vi "meth.PushErrorState.vi"(0 "class.GLue in":refnum<class "class.GLue.lvclass">, 11 "error in (no error)":errorcluster) -> (4 "class.GLue out":refnum<class "class.GLue.lvclass">, 8 "NumPushed":i32, 15 "error out":errorcluster)   [LabVIEW 2014, in "GLue.lvlib" / "class.GLue.lvclass"]
uses:
  class.GLue.lvclass
  class.GLue.lvclass/class.GLue.ctl
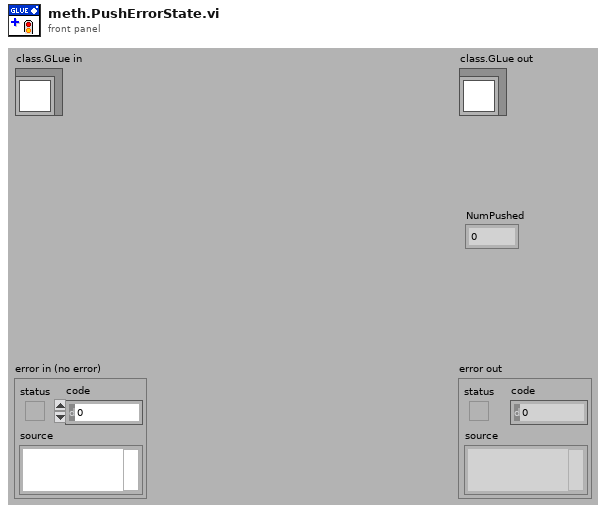
[diagram p1: front panel]
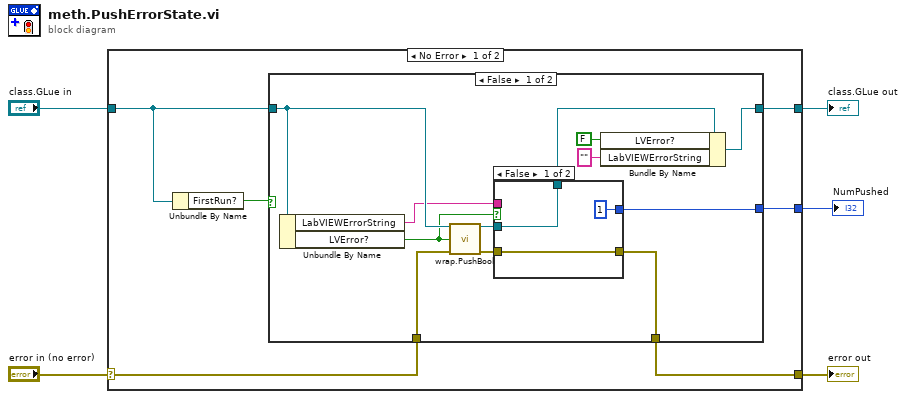
[diagram p0: block diagram]
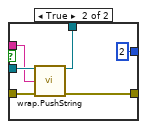
[diagram p2: hidden frame]
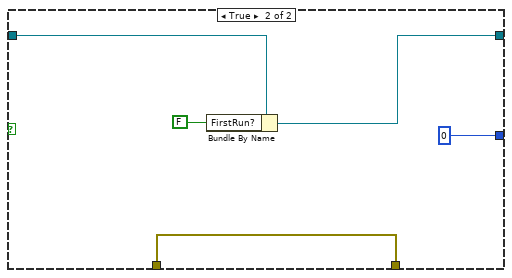
[diagram p3: hidden frame]
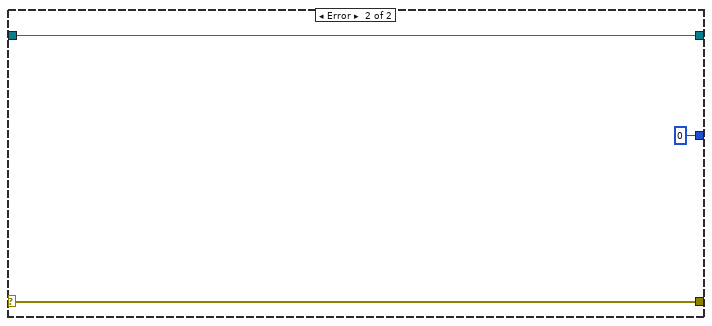
[diagram p4: hidden frame]
diagram:
  n1 = case shown="No Error" "error in (no error)" {
    selector: "error in (no error)" -> [w10 w40]
    tunnel: [w9 w40] -> w4
    tunnel: [w11 w39] -> w2
    tunnel: "class.GLue in" -> [w8 w39]
    tunnel: [w6 0] -> w1
    frame No Error {
      n2 = Unbundle By Name(w8) -> ("FirstRun?"=w7:bool)
      n3 = case shown="False" w7 {
        tunnel: [w23 w34] -> w11
        tunnel: w8 -> [w22 w35]
        tunnel: w10 -> [w20 w37]
        tunnel: [w18 w37] -> w9
        tunnel: [w12 0] -> w6
        frame False {
          n4 = Unbundle By Name(w22) -> ("LabVIEWErrorString"=w15:string, "LVError?"=w13:bool)
          n5 = call "wrap.PushBool.vi"("class.GLue in"=w22, "Boolean"=w13, "error in (no error)"=w20) -> ("class.GLue out"=w17:refnum<class "class.GLue.lvclass">, "error out"=w19:errorcluster)  [unwired: 11 in]
          n6 = case shown="False" w13 {
            tunnel: w19 -> [w26 w32]
            tunnel: [w26 w31] -> w18
            tunnel: w17 -> [w25 w30]
            tunnel: [w25 w29] -> w16
            tunnel: w15 -> [_ w28]
            tunnel: [1 2] -> w12
            frame False {
            }
            frame True {
              n7 = call "wrap.PushString.vi"("class.GLue in"=w30, "String"=w28, "error in (no error)"=w32) -> ("class.GLue out"=w29:refnum<class "class.GLue.lvclass">, "error out"=w31:errorcluster)  [unwired: 11 in]
            }
          }
          n8 = Bundle By Name(cluster=w16, "LVError?"=FALSE, "LabVIEWErrorString"="") -> (w23:refnum<class "class.GLue.lvclass">)
        }
        frame True {
          n9 = Bundle By Name(cluster=w35, "FirstRun?"=FALSE) -> (w34:refnum<class "class.GLue.lvclass">)
        }
      }
    }
    frame Error {
    }
  }
  "error out" <- w4
  "class.GLue out" <- w2
  "NumPushed" <- w1
